vi "Get_Validation_Inclusion_Type.vi"(8 "error in (no error)":errorcluster, 11 "AB_SourceDistribution in":refnum<class "AB_SourceDistribution.lvclass">) -> (0 "error out":errorcluster, 2 "sourceInclusion":T1=enum."TopLevel", 3 "AB_SourceDistribution out":refnum<class "AB_SourceDistribution.lvclass">)   [LabVIEW 2020, in "AB_SourceDistribution.lvclass"]
uses:
  <vilib>/AppBuilder/AB_Classes/SourceDistribution/AB_SourceDistribution.lvclass
  <vilib>/AppBuilder/AB_Source_Inclusion.ctl
  <vilib>/AppBuilder/AB_Classes/SourceDistribution/AB_SourceDistribution.lvclass/AB_SourceDistribution.ctl
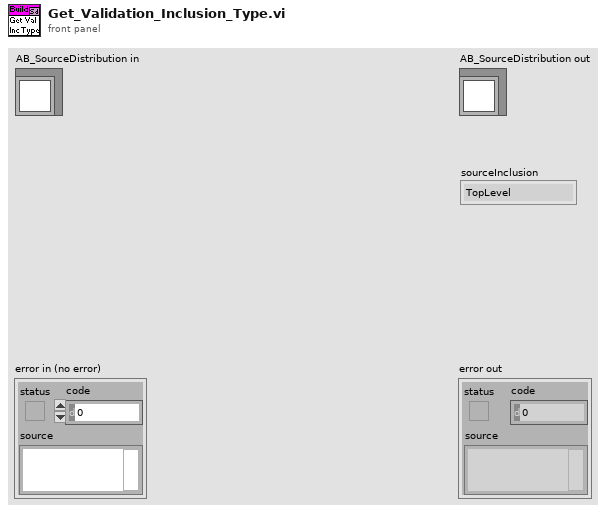
[diagram p1: front panel]
types:
  T1 = typedef "AB_Source_Inclusion.ctl" = enum16{"IncludeIfReferenced", "Include", "Exclude", "TopLevel"}
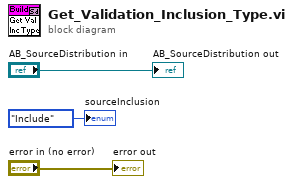
[diagram p0: block diagram]
diagram:
  "error out" <- "error in (no error)"
  "AB_SourceDistribution out" <- "AB_SourceDistribution in"
  "sourceInclusion" <- AB_Source_Inclusion."Include" ("sourceInclusion")
